vi "COM Error Checker.vi"(8 "error in (no error)":errorcluster, 10 "Command":string, 11 "Response":string) -> (0 "error out":errorcluster, 3 "Response":string)   [LabVIEW 2019, in "KH7008.lvlib"]
uses:
  KH7008.lvlib
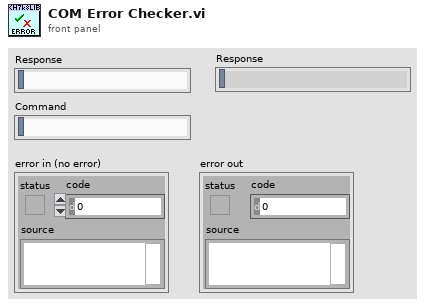
[diagram p1: front panel]
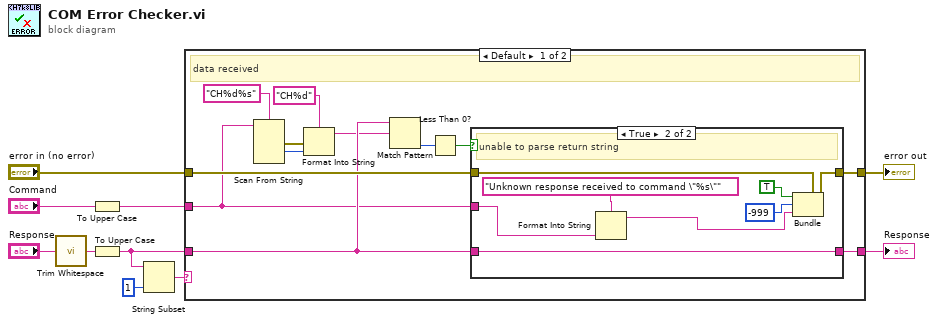
[diagram p0: block diagram]
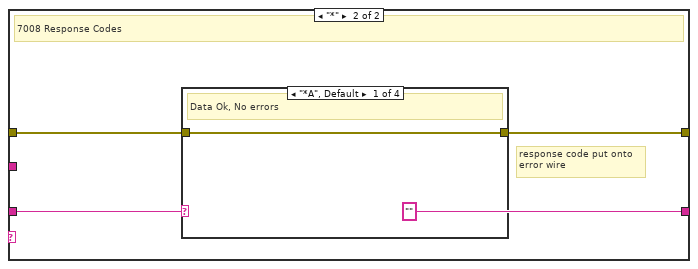
[diagram p3: hidden frame]
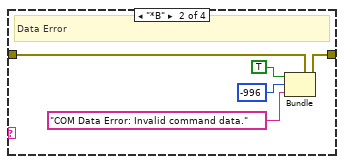
[diagram p4: hidden frame]
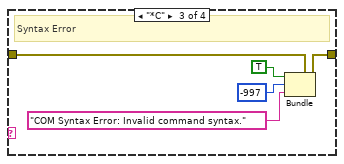
[diagram p5: hidden frame]
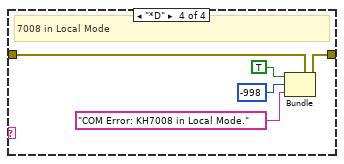
[diagram p6: hidden frame]
diagram:
  n1 = call <vilib>:"Trim Whitespace.vi"("string"="Response") -> ("trimmed string"=w5:string)  [unwired: 1 in]
  n2 = To Upper Case(1:"Command") -> (0:w1:string)
  n3 = To Upper Case(1:w5) -> (0:w3:string)
  n4 = String Subset(string=w3, length (rest)=1 ("length (rest)")) -> (substring=w6:string)  [unwired: 1 in]
  n5 = case shown="Default" w6 {
    tunnel: [w20 w36] -> w10
    tunnel: "error in (no error)" -> [w21 w35]
    tunnel: w3 -> [w18 w34]
    tunnel: [w17 "" ("trimmed string")] -> w4
    tunnel: w1 -> [w16 _]
    frame Default {
      # "data received"
      n6 = Scan From String(format string="CH%d%s", input string=w16) -> (error out=w14:errorcluster, output 1=w13:i32)  [unwired: 5 in, 2 out]
      n7 = Format Into String(format string="CH%d", error in=w14, w13) -> (resulting string=w11:string)  [unwired: 1 in, 1 out]
      n8 = Match Pattern(string=w18, regular expression=w11) -> (offset past match=w22:i32)  [unwired: 1 in, 3 out]
      n9 = Less Than 0?(x=w22) -> (x < 0?=w19:bool)
      n10 = case shown="True" w19 {
        tunnel: w21 -> [w24 w30]
        tunnel: [w24 w29] -> w20
        tunnel: w18 -> [w23 w28]
        tunnel: [w23 w28] -> w17
        tunnel: w16 -> [_ w26]
        frame False {
          # "Data Ok, No errors"
        }
        frame True {
          # "unable to parse return string"
          n11 = Format Into String(format string="Unknown response received to command \"%s\"" ("source"), w26) -> (resulting string=w25:string)  [unwired: 2 in, 1 out]
          n12 = Bundle(cluster=w30, "status"=TRUE, "code"=-999, "source"=w25) -> (w29:errorcluster)
        }
      }
    }
    frame "*" {
      # "response code put onto\nerror wire"
      # "7008 Response Codes"
      n13 = case shown="\"*A\", Default" w34 {
        tunnel: w35 -> [w37 w42 w47 w52]
        tunnel: [w37 w38 w43 w48] -> w36
        frame "*A", Default {
          # "Data Ok, No errors"
        }
        frame "*B" {
          # "Data Error"
          n14 = Bundle(cluster=w42, "status"=TRUE, "code"=-996, "source"="COM Data Error: Invalid command data.") -> (w38:errorcluster)
        }
        frame "*C" {
          # "Syntax Error"
          n15 = Bundle(cluster=w47, "status"=TRUE, "code"=-997, "source"="COM Syntax Error: Invalid command syntax.") -> (w43:errorcluster)
        }
        frame "*D" {
          # "7008 in Local Mode"
          n16 = Bundle(cluster=w52, "status"=TRUE, "code"=-998, "source"="COM Error: KH7008 in Local Mode.") -> (w48:errorcluster)
        }
      }
    }
  }
  "Response" <- w4
  "error out" <- w10
